vi "Colormap3DPlot.vi"(9 "Map Selector":T1(ring), 10 "Z matrix":i32[][](array[numeric]), 11 "Control in":refnum<vi>) -> ()   [LabVIEW 2020]
uses:
  <vilib>/Native 3D Graph/xcontrol/3DPC_SurfacePlot.xctl
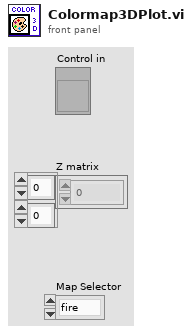
[diagram p1: front panel]
types:
  T1 = enum16{"fire", "rainbow", "gray", "inverse gray", "ice", "original"}
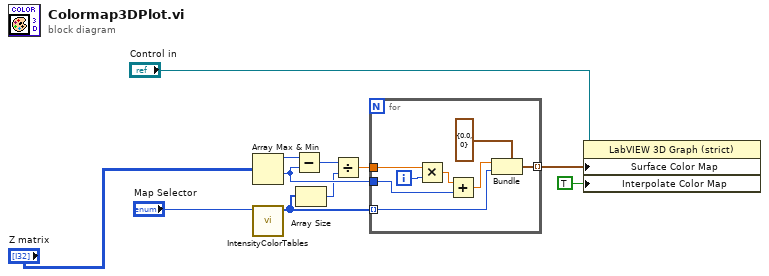
[diagram p0: block diagram]
diagram:
  n1 = Array Max & Min(array="Z matrix") -> (max value=w4:i32, min value=w9:i32)  [unwired: 2 out]
  n2 = call "IntensityColorTables.vi"("Map Selector"="Map Selector") -> ("Color Map Array"=w7:u32[])  [unwired: 10 in]
  n3 = Subtract(x=w4, y=w9) -> (x-y=w5:i32)
  n4 = Array Size(array=w7) -> (size(s)=w6:i32)
  n5 = Divide(x=w5, y=w6) -> (x/y=w8:dbl)
  n6 = for {
    tunnel: w7 -> [w18] mode=indexing
    tunnel: [w17] -> w2 mode=indexing
    tunnel: w8 -> [w16]
    tunnel: w9 -> [w14]
    i -> [w15]
    n7 = Multiply(x=w16, y=w15) -> (x*y=w13:dbl)
    n8 = Add(x=w13, y=w14) -> (x+y=w12:dbl)
    n9 = Bundle(cluster=cluster{dbl, u32} {0.0, 0} ("Plots:Surface Color Map"), w12, w18) -> (w17:cluster{dbl, u32})
  }
  n10 = property on="Property Node" class="LabVIEW 3D Graph (strict)"(reference="Control in", "Surface Color Map"=w2, "Interpolate Color Map"=TRUE) -> ()  [unwired: 1 in, 2 out]
